vi "MT Apply Pulse Shaping Filter (Offset PSK).vi"(0 "symbols":cdb[](array[numeric]) format="%.2f", 5 "pulse shaping filter coefficients":dbl[](array[numeric]) format="%.2f", 7 "samples per symbol (16)":i32=16, 9 "symbol rate (Hz)":dbl=1.0, 11 "error in (no error)":errorcluster, 13 "reset? (T)":bool=TRUE) -> (4 "output complex waveform":T1={"t0"=0.0, "dt"=1.0, "Y"=[]} {"Y" format="%.3f"; "dt" format="%^.2e"; "t0" format="%.4f"}, 15 "error out":errorcluster)   [LabVIEW 2020, in "niDMT.lvlib"]
doc: "This polymorphic instance applies a pulse-shaping filter to an input stream comprised of offset PSK-modulated symbols. The VI shifts the Q-phase baseband data by ½ symbol relative to the I-phase baseband data, so the first Q-symbol lasts for the duration of 1.5 symbol periods.\n\n<B>NOTE:</B> Use the generic instance of this VI for nonoffset PSK-modulated signals."
uses:
  <vilib>/addons/Modulation/niDMT.lvlib
  <vilib>/addons/Modulation/Analog/controls/Complex Data Waveform.ctl
  <vilib>/addons/Modulation/niAMT.lvlib
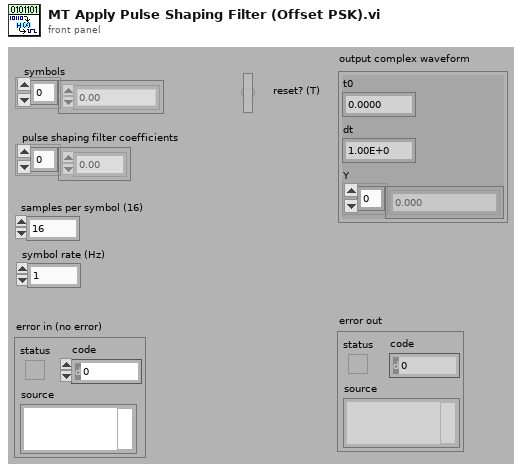
[diagram p1: front panel]
types:
  T1 = typedef "niAMT.lvlib/Complex Data Waveform.ctl" = cluster{"t0":dbl, "dt":dbl, "Y":cdb[]}
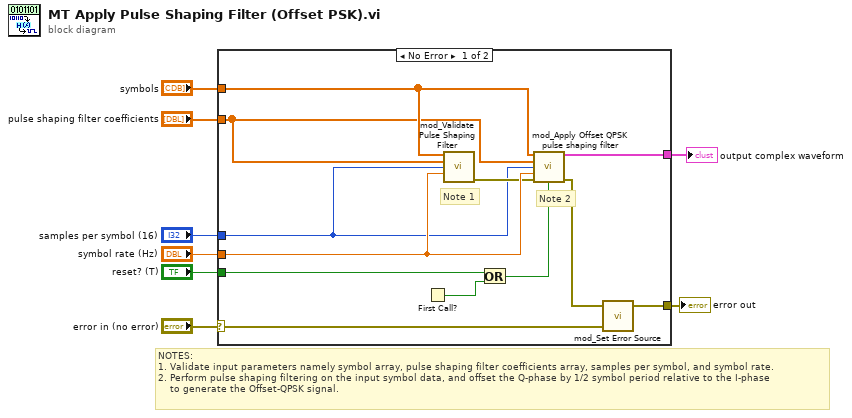
[diagram p0: block diagram]
diagram:
  # "NOTES:\n1. Validate input parameters namely symbol array, pulse shaping filter coefficients array, samples per symbol, and symbol rate.\n2. Perform pulse shaping filtering on the input symbol data, and offset the Q-phase by 1/2 symbol period relative to the I-phase\n    to generate the Offset-QPSK signal."
  n1 = case shown="No Error" "error in (no error)" {
    selector: "error in (no error)" -> [w11 w21]
    tunnel: "symbols" -> [w16 _]
    tunnel: "pulse shaping filter coefficients" -> [w15 _]
    tunnel: "samples per symbol (16)" -> [w12 _]
    tunnel: "symbol rate (Hz)" -> [w14 _]
    tunnel: "reset? (T)" -> [w20 _]
    tunnel: [w9 w21] -> w1
    tunnel: [w17 _] -> w2
    frame No Error {
      # "Note 2"
      # "Note 1"
      n2 = First Call?() -> (First Call?: T/F=w19:bool)
      n3 = call <vilib>:"mod_Validate Pulse Shaping Filter.vi"("symbols"=w16, "pulse shaping filter coefficients"=w15, "samples per symbol (16)"=w12, "symbol Rate, Hz"=w14) -> ("error out"=w13:errorcluster)  [unwired: 11 out]
      n4 = Or(x=w20, y=w19) -> (x .or. y?=w18:bool)
      n5 = call <vilib>:"mod_Apply Offset QPSK pulse shaping filter.vi"("symbols"=w16, "pulse shaping filter coefficients"=w15, "samples per symbol (16)"=w12, "symbol rate"=w14, "error in (no error)"=w13, "reset? (T)"=w18) -> ("output complex waveform"=w17:T1, "error out"=w10:errorcluster)  [unwired: 8 out]
      n6 = call <vilib>:"mod_Set Error Source.vi"("initial error in (no error)"=w11, "final error in (no error)"=w10) -> ("error out"=w9:errorcluster)  [unwired: 3 out]
    }
    frame Error {
    }
  }
  "error out" <- w1
  "output complex waveform" <- w2
